vi "getWIPDataByCustLotNo.vi"(8 "error out 2":errorcluster, 10 "Lotno":string="A141100029", 11 "connection reference":T1) -> (0 "error out":errorcluster, 1 "output array":string[][](array[string]), 2 "data":i32, 3 "connection reference 2":T1)   [LabVIEW 2012]
uses:
  <vilib>/addons/database/Connection.llb/Conn ObjectReference.ctl
  <vilib>/addons/database/Auxilliary.llb/DB Tools Cursor Type.ctl
  <vilib>/addons/database/Connection.llb/Conn Execute.vi
  <vilib>/addons/database/Recordset.llb/Rec Fetch Integer Data (R).vi
  <vilib>/addons/database/Recordset.llb/Rec Destroy - Connection.vi
  <vilib>/addons/database/Recordset.llb/Rec Fetch Recordset Data (R).vi
  <vilib>/addons/database/_DB Variant To Data/Database Variant To Data.xnode
  <vilib>/addons/database/NI_Database_API.lvlib
panel:
  out "concatenated string":string
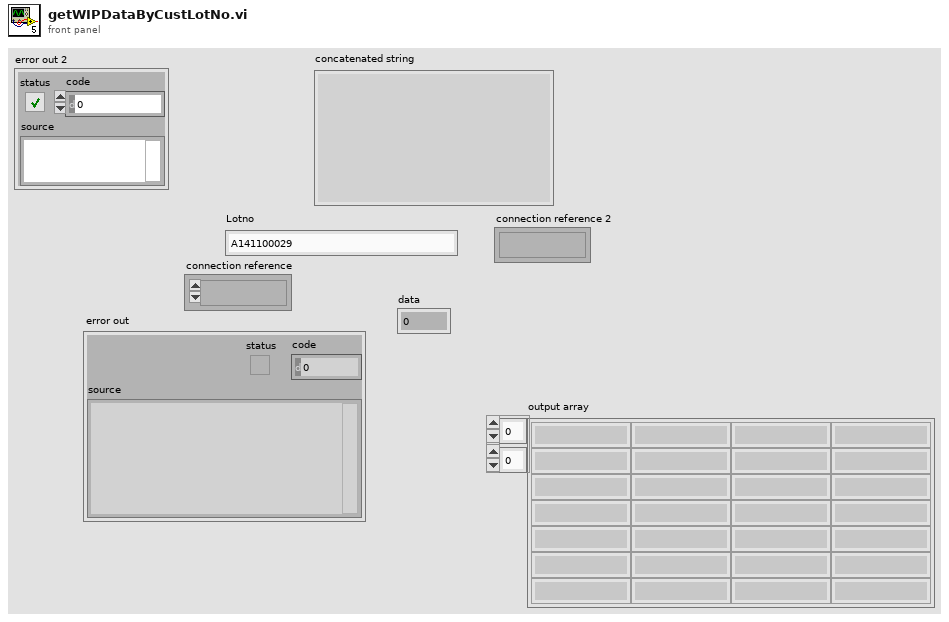
[diagram p1: front panel]
types:
  T1 = typedef "NI_Database_API.lvlib/Conn ObjectReference.ctl" = refnum<k1>
  T2 = typedef "NI_Database_API.lvlib/DB Tools Cursor Type.ctl" = enum16{"forward-only", "keyset", "dynamic", "static"}
  T3 = typedef "NI_Database_API.lvlib/Rec ObjectReference.ctl" = refnum<k1>
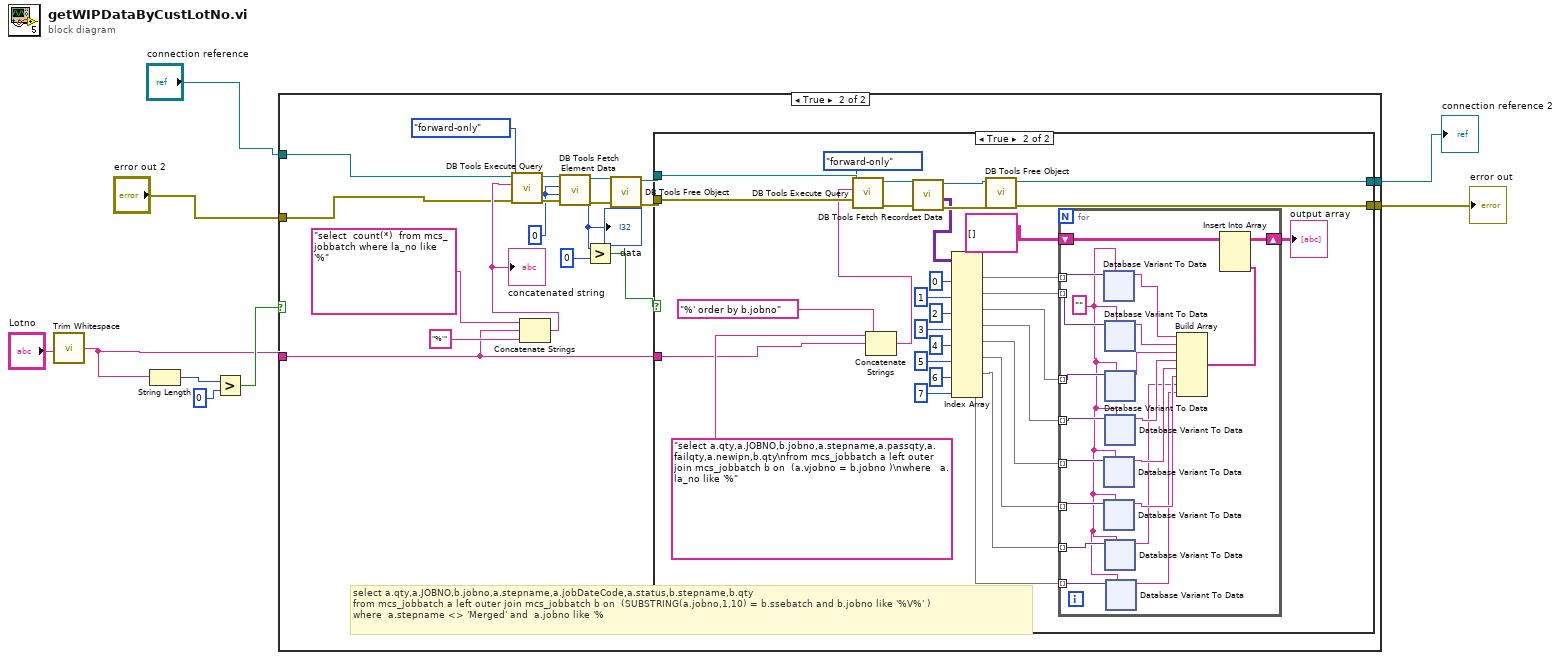
[diagram p0: block diagram]
diagram:
  n1 = call <vilib>:"Trim Whitespace.vi"("string"="Lotno") -> ("trimmed string"=w1:string)  [unwired: 1 in]
  n2 = String Length(string=w1) -> (length=w9:i32)
  n3 = Greater?(x=w9, y=0) -> (0:w7:bool)
  n4 = case shown="True" w7 {
    tunnel: w1 -> [_ w26]
    tunnel: "error out 2" -> [w10 w15]
    tunnel: "connection reference" -> [w11 w14]
    tunnel: [w11 w13] -> w3
    tunnel: [w10 w12] -> w4
    frame False {
    }
    frame True {
      w19 = 0
      # "select a.qty,a.JOBNO,b.jobno,a.stepname,a.jobDateCode,a.status,b.stepname,b.qty\nfrom mcs_jobbatch a left outer join mcs_jobbatch b on  (SUBSTRING(a.jobno,1,10) = b.ssebatch and b.jobno like '%V%' )\nwhere  a.stepname <> 'Merged' and  a.jobno like '%"
      n5 = Concatenate Strings("select  count(*)  from mcs_jobbatch where la_no like '%" ("string"), w26, "%'" ("string")) -> (w24:string)
      "concatenated string" <- w24
      n6 = call-poly <vilib>:"DB Tools Execute Query.vi"("error in (no error)"=w15, "cursor type"=DB_Tools_Cursor_Type."forward-only", "SQL query"=w24, "connection reference"=w14) -> ("error out"=w23:errorcluster, "recordset reference"=w22:T3)  [unwired: 4 in]
      n7 = call-poly <vilib>:"DB Tools Fetch Element Data.vi"("error in (no error)"=w23, "type"=w19, "column index"=w19, "recordset reference"=w22) -> ("error out"=w20:errorcluster, "data"=w18:i32, "recordset reference out"=w21:T3)  [unwired: 3 in]
      "data" <- w18
      n8 = Greater?(x=w18, y=0) -> (0:w16:bool)
      n9 = call-poly <vilib>:"DB Tools Free Object.vi"("error in (no error)"=w20, "recordset reference"=w21) -> ("error out"=w29:errorcluster, "connection reference"=w30:T1)  [unwired: 8 in]
      n10 = case shown="True" w16 {
        tunnel: w30 -> [w32 w64]
        tunnel: w29 -> [w31 w61]
        tunnel: w26 -> [_ w54]
        tunnel: [w32 w53] -> w13
        tunnel: [w31 w52] -> w12
        frame False {
        }
        frame True {
          n11 = Concatenate Strings("select a.qty,a.JOBNO,b.jobno,a.stepname,a.passqty,a.failqty,a.newipn,b.qty\nfrom mcs_jobbatch a left outer join mcs_jobbatch b on  (a.vjobno = b.jobno )\nwhere   a.la_no like '%" ("string"), w54, "%' order by b.jobno" ("string")) -> (w55:string)
          n12 = call-poly <vilib>:"DB Tools Execute Query.vi"("error in (no error)"=w61, "cursor type"=DB_Tools_Cursor_Type."forward-only", "SQL query"=w55, "connection reference"=w64) -> ("error out"=w60:errorcluster, "recordset reference"=w63:T3)  [unwired: 4 in]
          n13 = call-poly <vilib>:"DB Tools Fetch Recordset Data.vi"("error in (no error)"=w60, "recordset reference"=w63) -> ("error out"=w59:errorcluster, "recordset data"=w51:variant[][], "recordset reference out"=w62:T3)  [unwired: 3 in]
          n14 = Index Array(array=w51, index (col) #1=0 ("disabled index (col)"), index (col) #2=1 ("index (col)"), index (col) #3=2 ("index (col)"), index (col) #4=3 ("index (col)"), index (col) #5=4 ("index (col)"), index (col) #6=5 ("index (col)"), index (col) #7=6 ("index (col)"), index (col) #8=7 ("index (col)")) -> (element #1=w44:variant[], element #2=w43:variant[], element #3=w42:variant[], element #4=w41:variant[], element #5=w40:variant[], element #6=w39:variant[], element #7=w34:variant[], element #8=w33:variant[])  [unwired: 8 in]
          n15 = call-poly <vilib>:"DB Tools Free Object.vi"("error in (no error)"=w59, "recordset reference"=w62) -> ("error out"=w52:errorcluster, "connection reference"=w53:T1)  [unwired: 8 in]
          n16 = for {
            tunnel: w44 -> [w84] mode=indexing
            tunnel: w43 -> [w83] mode=indexing
            tunnel: w42 -> [w82] mode=indexing
            tunnel: w41 -> [w81] mode=indexing
            tunnel: w40 -> [w80] mode=indexing
            tunnel: w39 -> [w79] mode=indexing
            shift-right: [w71] -> w37
            shift-left: string[][] [] ("output array") -> [w70]
            tunnel: w34 -> [w69] mode=indexing
            tunnel: w33 -> [w67] mode=indexing
            w66 = ""
            n17 = xnode "Database Variant To Data"("database variant"=w84, "type"=w66) -> ("data"=w78:string)  [unwired: 1 in, 1 out]
            n18 = xnode "Database Variant To Data"("database variant"=w80, "type"=w66) -> ("data"=w74:string)  [unwired: 1 in, 1 out]
            n19 = xnode "Database Variant To Data"("database variant"=w79, "type"=w66) -> ("data"=w73:string)  [unwired: 1 in, 1 out]
            n20 = xnode "Database Variant To Data"("database variant"=w83, "type"=w66) -> ("data"=w77:string)  [unwired: 1 in, 1 out]
            n21 = xnode "Database Variant To Data"("database variant"=w82, "type"=w66) -> ("data"=w76:string)  [unwired: 1 in, 1 out]
            n22 = xnode "Database Variant To Data"("database variant"=w81, "type"=w66) -> ("data"=w75:string)  [unwired: 1 in, 1 out]
            n23 = xnode "Database Variant To Data"("database variant"=w69, "type"=w66) -> ("data"=w68:string)  [unwired: 1 in, 1 out]
            n24 = xnode "Database Variant To Data"("database variant"=w67, "type"=w66) -> ("data"=w65:string)  [unwired: 1 in, 1 out]
            n25 = Build Array(w78, w77, w76, w75, w74, w73, w68, w65) -> (w72:string[])
            n26 = Insert Into Array(array=w70, new element=w72) -> (w71:string[][])  [unwired: 2 in]
          }
          "output array" <- w37
        }
      }
    }
  }
  "connection reference 2" <- w3
  "error out" <- w4
